vi "Signal_Name_Conver.vi"(11 "signal_array":T1[](array[typedef])) -> (3 "Signals":string[][](array[string]))   [LabVIEW 2014]
uses:
  Typedef/CAN/TCANSignal.ctl
  Typedef/LIN/TLINSignal.ctl
  Typedef/FlexRay/TFlexRaySignal.ctl
  Typedef/TDBSignalProperties.ctl
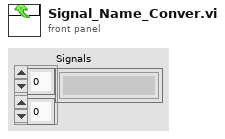
[diagram p1: front panel]
types:
  T1 = typedef "TDBSignalProperties.ctl" = cluster{"FDBIndex":i32, "FECUIndex":i32, "FFrameIndex":i32, "FSignalIndex":i32, "FIsTx":u8, "FReserved1":u8, "FReserved2":u8, "FReserved3":u8, "TSignalType":i32, "TCANSignal":T2, "TLINSignal":T3, "TFlexRaySignal":T4, "FParentFrameId":i32, "FInitValue":dbl, "FName":cluster{"数值":u64, "数值 2":u64, "数值 3":u64, "数值 4":u64, "数值 5":u64, "数值 6":u64, "数值 7":u64, "数值 8":u64, "数值 9":u64, "数值 10":u64, "数值 11":u64, "数值 12":u64, "数值 13":u64, "数值 14":u64, "数值 15":u64, "数值 16":u64, "数值 17":u64, "数值 18":u64, "数值 19":u64, "数值 20":u64, "数值 21":u64, "数值 22":u64, "数值 23":u64, "数值 24":u64, "数值 25":u64, "数值 26":u64, "数值 27":u64, "数值 28":u64, "数值 29":u64, "数值 30":u64, "数值 31":u64, "数值 32":u64, "数值 33":u64, "数值 34":u64, "数值 35":u64, "数值 36":u64, "数值 37":u64, "数值 38":u64, "数值 39":u64, "数值 40":u64, "数值 41":u64, "数值 42":u64, "数值 43":u64, "数值 44":u64, "数值 45":u64, "数值 46":u64, "数值 47":u64, "数值 48":u64, "数值 49":u64, "数值 50":u64, "数值 51":u64, "数值 52":u64, "数值 53":u64, "数值 54":u64, "数值 55":u64, "数值 56":u64, "数值 57":u64, "数值 58":u64, "数值 59":u64, "数值 60":u64, "数值 61":u64, "数值 62":u64, "数值 63":u64, "数值 64":u64}, "FComment":cluster{"数值":u64, "数值 2":u64, "数值 3":u64, "数值 4":u64, "数值 5":u64, "数值 6":u64, "数值 7":u64, "数值 8":u64, "数值 9":u64, "数值 10":u64, "数值 11":u64, "数值 12":u64, "数值 13":u64, "数值 14":u64, "数值 15":u64, "数值 16":u64, "数值 17":u64, "数值 18":u64, "数值 19":u64, "数值 20":u64, "数值 21":u64, "数值 22":u64, "数值 23":u64, "数值 24":u64, "数值 25":u64, "数值 26":u64, "数值 27":u64, "数值 28":u64, "数值 29":u64, "数值 30":u64, "数值 31":u64, "数值 32":u64, "数值 33":u64, "数值 34":u64, "数值 35":u64, "数值 36":u64, "数值 37":u64, "数值 38":u64, "数值 39":u64, "数值 40":u64, "数值 41":u64, "数值 42":u64, "数值 43":u64, "数值 44":u64, "数值 45":u64, "数值 46":u64, "数值 47":u64, "数值 48":u64, "数值 49":u64, "数值 50":u64, "数值 51":u64, "数值 52":u64, "数值 53":u64, "数值 54":u64, "数值 55":u64, "数值 56":u64, "数值 57":u64, "数值 58":u64, "数值 59":u64, "数值 60":u64, "数值 61":u64, "数值 62":u64, "数值 63":u64, "数值 64":u64}}
  T2 = typedef "TCANSignal.ctl" = cluster{"FCANSgnType":u8, "FIsIntel":u8, "FStartBit":i32, "FLength":i32, "FFactor":dbl, "FOffset":dbl}
  T3 = typedef "TLINSignal.ctl" = cluster{"FLINSgnType":u8, "FIsIntel":u8, "FStartBit":i32, "FLength":i32, "FFactor":dbl, "FOffset":dbl}
  T4 = typedef "TFlexRaySignal.ctl" = cluster{"FFRSgnType":u8, "FCompuMethod":u8, "FReserved":u8, "FIsIntel":u8, "FStartBit":i32, "FUpdateBit":i32, "FLength":i32, "FFactor":dbl, "FOffset":dbl, "FActualStartBit":i32, "FActualUpdateBit":i32}
  T5 = cluster{"数值":u64, "数值 2":u64, "数值 3":u64, "数值 4":u64, "数值 5":u64, "数值 6":u64, "数值 7":u64, "数值 8":u64, "数值 9":u64, "数值 10":u64, "数值 11":u64, "数值 12":u64, "数值 13":u64, "数值 14":u64, "数值 15":u64, "数值 16":u64, "数值 17":u64, "数值 18":u64, "数值 19":u64, "数值 20":u64, "数值 21":u64, "数值 22":u64, "数值 23":u64, "数值 24":u64, "数值 25":u64, "数值 26":u64, "数值 27":u64, "数值 28":u64, "数值 29":u64, "数值 30":u64, "数值 31":u64, "数值 32":u64, "数值 33":u64, "数值 34":u64, "数值 35":u64, "数值 36":u64, "数值 37":u64, "数值 38":u64, "数值 39":u64, "数值 40":u64, "数值 41":u64, "数值 42":u64, "数值 43":u64, "数值 44":u64, "数值 45":u64, "数值 46":u64, "数值 47":u64, "数值 48":u64, "数值 49":u64, "数值 50":u64, "数值 51":u64, "数值 52":u64, "数值 53":u64, "数值 54":u64, "数值 55":u64, "数值 56":u64, "数值 57":u64, "数值 58":u64, "数值 59":u64, "数值 60":u64, "数值 61":u64, "数值 62":u64, "数值 63":u64, "数值 64":u64}
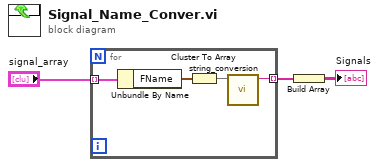
[diagram p0: block diagram]
diagram:
  n1 = for {
    tunnel: "signal_array" -> [w7] mode=indexing
    tunnel: [w4] -> w2 mode=indexing
    n2 = Unbundle By Name(w7) -> ("FName"=w5:T5)
    n3 = Cluster To Array(cluster=w5) -> (array=w6:u64[])
    n4 = call "string_conversion.vi"("FName"=w6) -> ("string"=w4:string)  [unwired: 10 in]
  }
  n5 = Build Array(w2) -> (→"Signals":string[][])
